vi "VI for temp, humidity, moisture and pH with power supply control final.vi"() -> ()   [LabVIEW 2022 SP3]
uses:
  <vilib>/DAQmx/read.llb/DAQmx Read (Analog 1D DBL NChan 1Samp).vi
  <vilib>/DAQmx/write.llb/DAQmx Write (Digital Bool 1Line 1Point).vi
  <vilib>/DAQmx/create/channels.llb/DAQmx Create Channel (AI-Voltage-Basic).vi
  <vilib>/DAQmx/create/channels.llb/DAQmx Create Channel (DO-Digital Output).vi
  <vilib>/DAQmx/miscellaneous.llb/DAQmx Fill In Error Info.vi
panel:
  out "pH meter":dbl(knob) scale=0.0..14.0
  out "Moisture":dbl(knob) scale=0.0..100.0
  out "Temperature":dbl(knob) scale=0.0..40.0
  out "Humidity":dbl(knob) scale=0.0..100.0
  in  "LED to notify pH level is out of range":tag
  in  "Trigger pump to water the plant":tag
  in  "VISA resource name - for close channel":refnum<visa-resource-name>
  in  "VISA resource name - for open channel":refnum<visa-resource-name>
  in  "Fan to reduce temperature":tag
  in  "Humidifier to increase humidity":tag
  in  "Fan to reduce humidity":tag
  in  "physical channels":tag
  in  "stop":bool
  out "voltage for humidity":dbl
  out "Humidity level":dbl
  out "Temperature level":dbl
  out "voltage for temperature":dbl
  out "voltage for moisture sensor":dbl
  out "voltage for pH level":dbl
  out "Moisture level":dbl
  out "pH level":dbl
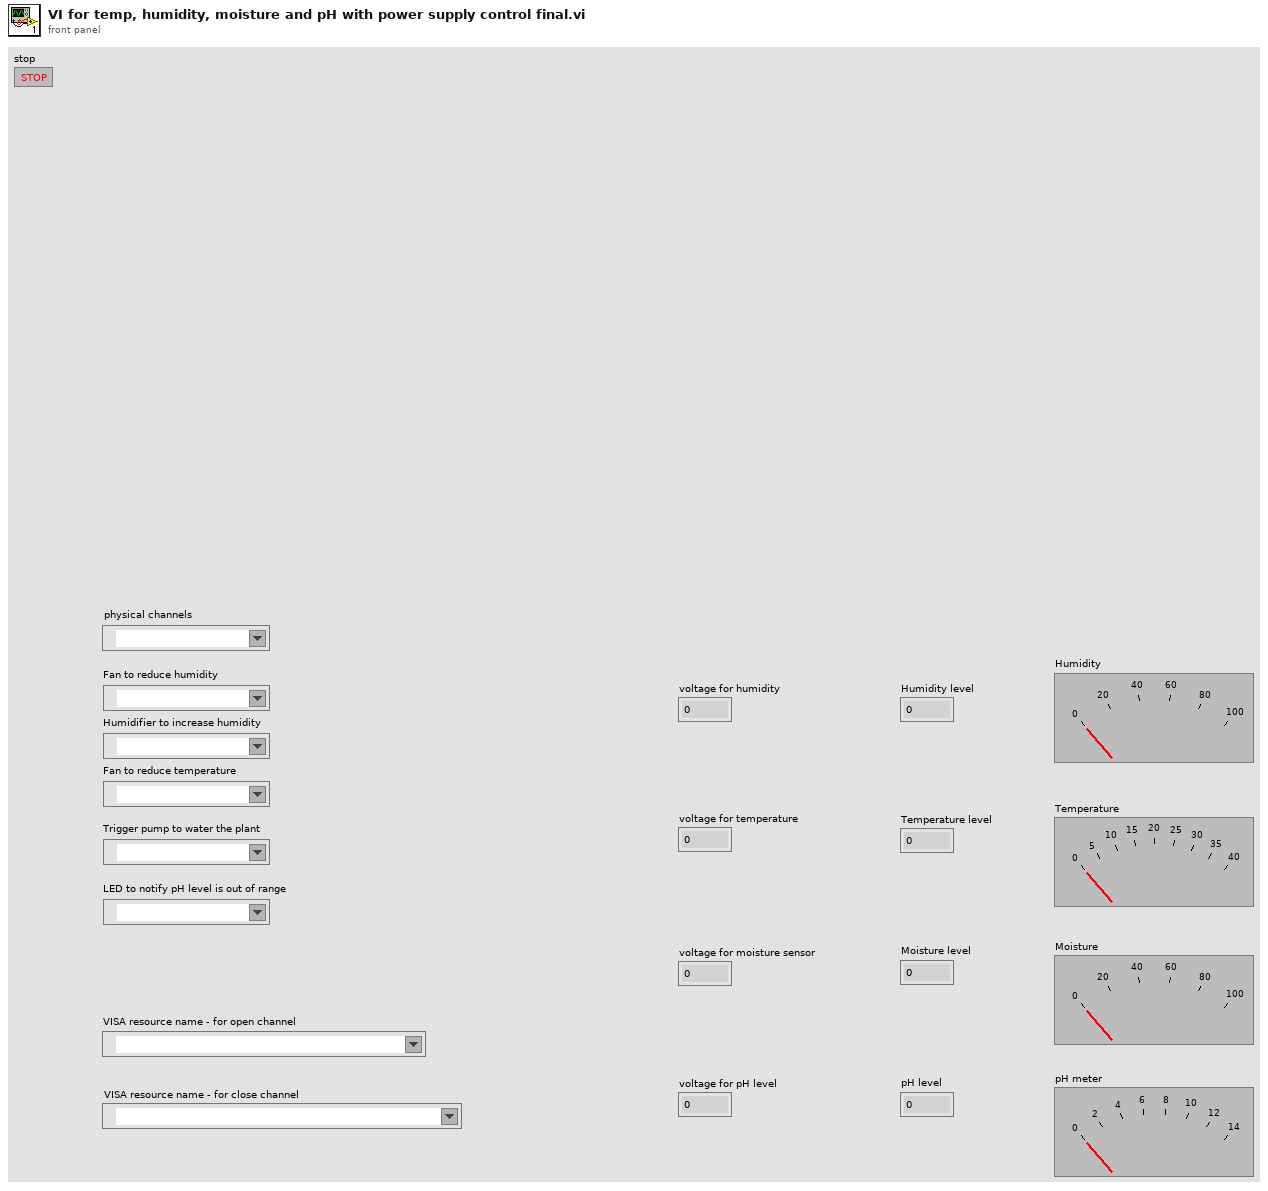
[diagram p1: front panel]
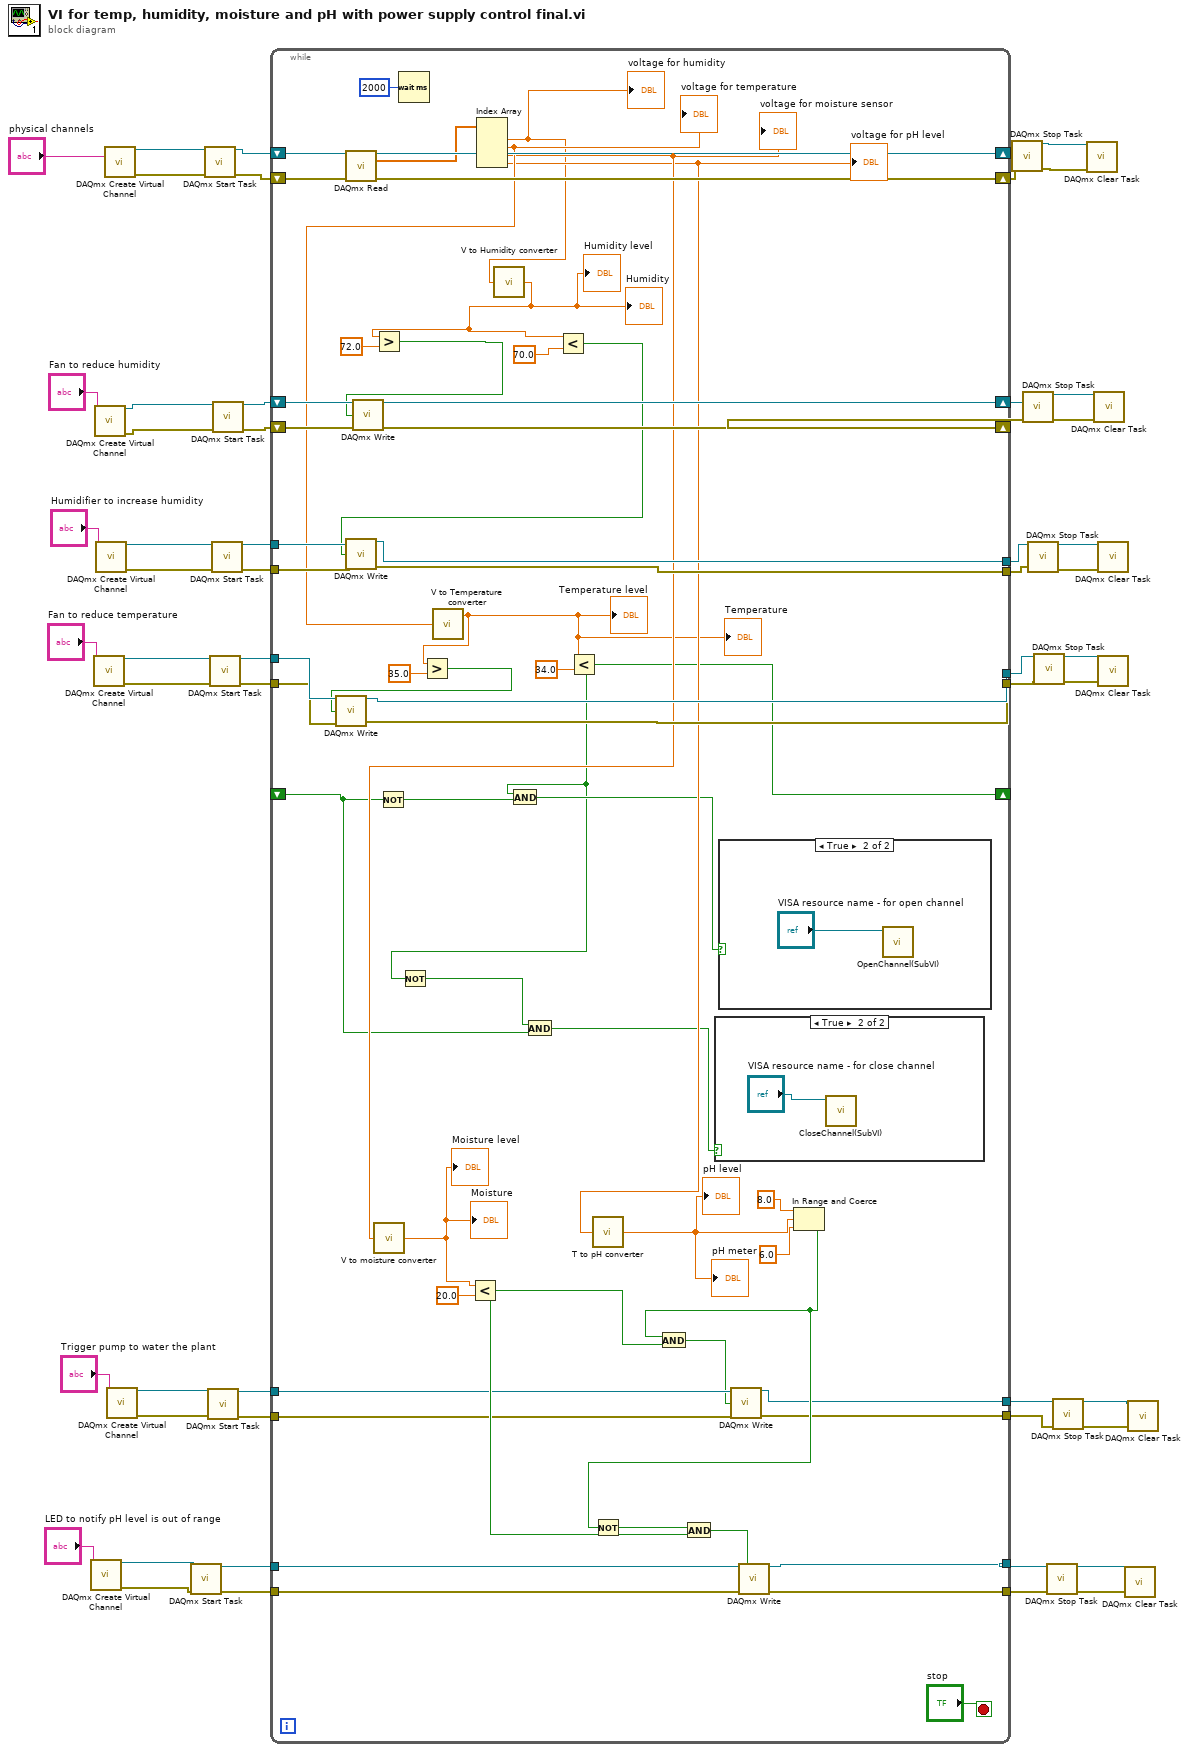
[diagram p0: block diagram]
diagram:
  n1 = call-poly <vilib>:"DAQmx Create Virtual Channel.vi"("lines"="LED to notify pH level is out of range") -> ("task out"=w9:refnum<k21>, "error out"=w5:errorcluster)  [unwired: 13 in]
  n2 = call-poly <vilib>:"DAQmx Create Virtual Channel.vi"("lines"="Fan to reduce temperature") -> ("task out"=w27:refnum<k21>, "error out"=w26:errorcluster)  [unwired: 13 in]
  n3 = call-poly <vilib>:"DAQmx Create Virtual Channel.vi"("lines"="Fan to reduce humidity") -> ("task out"=w46:refnum<k21>, "error out"=w42:errorcluster)  [unwired: 13 in]
  n4 = call-poly <vilib>:"DAQmx Create Virtual Channel.vi"("lines"="Humidifier to increase humidity") -> ("task out"=w36:refnum<k21>, "error out"=w35:errorcluster)  [unwired: 13 in]
  n5 = call-poly <vilib>:"DAQmx Create Virtual Channel.vi"("physical channels"="physical channels") -> ("task out"=w54:refnum<k21>, "error out"=w50:errorcluster)  [unwired: 13 in]
  n6 = call-poly <vilib>:"DAQmx Create Virtual Channel.vi"("lines"="Trigger pump to water the plant") -> ("task out"=w18:refnum<k21>, "error out"=w14:errorcluster)  [unwired: 13 in]
  n7 = call <vilib>:"DAQmx Start Task.vi"("task/channels in"=w9, "error in"=w5) -> ("task out"=w8:refnum<k21>, "error out"=w4:errorcluster)  [unwired: 12 in]
  n8 = call <vilib>:"DAQmx Start Task.vi"("task/channels in"=w54, "error in"=w50) -> ("task out"=w53:refnum<k21>, "error out"=w49:errorcluster)  [unwired: 12 in]
  n9 = call <vilib>:"DAQmx Start Task.vi"("task/channels in"=w18, "error in"=w14) -> ("task out"=w17:refnum<k21>, "error out"=w13:errorcluster)  [unwired: 12 in]
  n10 = call <vilib>:"DAQmx Start Task.vi"("task/channels in"=w27, "error in"=w26) -> ("task out"=w24:refnum<k21>, "error out"=w23:errorcluster)  [unwired: 12 in]
  n11 = call <vilib>:"DAQmx Start Task.vi"("task/channels in"=w36, "error in"=w35) -> ("task out"=w34:refnum<k21>, "error out"=w33:errorcluster)  [unwired: 12 in]
  n12 = call <vilib>:"DAQmx Start Task.vi"("task/channels in"=w46, "error in"=w42) -> ("task out"=w45:refnum<k21>, "error out"=w41:errorcluster)  [unwired: 12 in]
  n13 = while {
    shift-right: [w109] -> w52
    shift-left: w53 -> [w110]
    shift-right: [w107] -> w48
    shift-left: w49 -> [w108]
    shift-right: [w105] -> w44
    shift-left: w45 -> [w106]
    shift-right: [w103] -> w40
    shift-left: w41 -> [w104]
    tunnel: w34 -> [w98]
    tunnel: w33 -> [w97]
    tunnel: [w96] -> w32
    tunnel: [w95] -> w31
    tunnel: w24 -> [w94]
    tunnel: w23 -> [w93]
    tunnel: [w92] -> w22
    tunnel: [w91] -> w21
    shift-right: [w81] -> _
    shift-left: _ -> [w63]
    tunnel: w17 -> [w74]
    tunnel: [w73] -> w16
    tunnel: w13 -> [w72]
    tunnel: [w71] -> w12
    tunnel: w8 -> [w69]
    tunnel: [w68] -> w7
    tunnel: w4 -> [w67]
    tunnel: [w66] -> w3
    stop <- "stop" stop-if-true
    n14 = call-poly <vilib>:"DAQmx Read.vi"("task/channels in"=w110, "error in"=w108) -> ("task out"=w109:refnum<k21>, "data"=w100:dbl[], "error out"=w107:errorcluster)  [unwired: 11 in]
    n15 = Not(x=w63) -> (.not. x?=w64:bool)
    n16 = Wait (ms)(milliseconds to wait=u32 2000) -> ()  [unwired: 1 out]
    n17 = Index Array(array=w100) -> (element #1=w78:dbl, element #2=w90:dbl, element #3=w86:dbl, element #4=w83:dbl)  [unwired: 4 in]
    "voltage for humidity" <- w78
    "voltage for temperature" <- w90
    "voltage for moisture sensor" <- w86
    "voltage for pH level" <- w83
    n18 = call "V to moisture converter.vi"("Waveform"=w86) -> ("Numeric"=w56:dbl)
    "Moisture level" <- w56
    "Moisture" <- w56
    n19 = call "V to Temperature converter.vi"("Waveform"=w90) -> ("Numeric"=w57:dbl)
    "Temperature level" <- w57
    "Temperature" <- w57
    n20 = Greater?(x=w57, y=35.0) -> (0:w59:bool)
    n21 = call-poly <vilib>:"DAQmx Write.vi"("task/channels in"=w94, "data"=w59, "error in"=w93) -> ("task out"=w92:refnum<k21>, "error out"=w91:errorcluster)  [unwired: 10 in, 1 out]
    n22 = Less?(x=w56, y=20.0) -> (x < y?=w75:bool)
    n23 = call "V to Humidity converter.vi"("Waveform"=w78) -> ("Numeric"=w58:dbl)
    "Humidity level" <- w58
    "Humidity" <- w58
    n24 = Greater?(x=w58, y=72.0) -> (0:w60:bool)
    n25 = call-poly <vilib>:"DAQmx Write.vi"("task/channels in"=w106, "data"=w60, "error in"=w104) -> ("task out"=w105:refnum<k21>, "error out"=w103:errorcluster)  [unwired: 10 in, 1 out]
    n26 = Less?(x=w58, y=70.0) -> (x < y?=w61:bool)
    n27 = call-poly <vilib>:"DAQmx Write.vi"("task/channels in"=w98, "data"=w61, "error in"=w97) -> ("task out"=w96:refnum<k21>, "error out"=w95:errorcluster)  [unwired: 10 in, 1 out]
    n28 = Less?(x=w57, y=34.0) -> (x < y?=w81:bool)
    n29 = Not(x=w81) -> (.not. x?=w80:bool)
    n30 = And(x=w81, y=w64) -> (x .and. y?=w82:bool)
    n31 = And(x=w80, y=w63) -> (x .and. y?=w79:bool)
    n32 = call "T to pH converter.vi"("Waveform"=w83) -> ("Numeric"=w55:dbl)
    "pH level" <- w55
    "pH meter" <- w55
    n33 = case shown="True" w79 {
      frame False {
      }
      frame True {
        n34 = call "CloseChannel(SubVI).vi"("VISA Refnum in"="VISA resource name - for close channel") -> ()  [unwired: 11 in]
      }
    }
    n35 = case shown="True" w82 {
      frame False {
      }
      frame True {
        n36 = call "OpenChannel(SubVI).vi"("VISA Refnum in"="VISA resource name - for open channel") -> ()  [unwired: 11 in]
      }
    }
    n37 = In Range and Coerce(upper limit=8.0, x=w55, lower limit=6.0) -> (In Range?=w77:bool)  [unwired: 1 out]
    n38 = Not(x=w77) -> (.not. x?=w76:bool)
    n39 = And(x=w77, y=w75) -> (x .and. y?=w70:bool)
    n40 = And(x=w76, y=w75) -> (x .and. y?=w65:bool)
    n41 = call-poly <vilib>:"DAQmx Write.vi"("task/channels in"=w74, "data"=w70, "error in"=w72) -> ("task out"=w73:refnum<k21>, "error out"=w71:errorcluster)  [unwired: 10 in, 1 out]
    n42 = call-poly <vilib>:"DAQmx Write.vi"("task/channels in"=w69, "data"=w65, "error in"=w67) -> ("task out"=w68:refnum<k21>, "error out"=w66:errorcluster)  [unwired: 10 in, 1 out]
  }
  n43 = call <vilib>:"DAQmx Stop Task.vi"("task/channels in"=w52, "error in"=w48) -> ("task out"=w51:refnum<k21>, "error out"=w47:errorcluster)  [unwired: 12 in]
  n44 = call <vilib>:"DAQmx Stop Task.vi"("task/channels in"=w44, "error in"=w40) -> ("task out"=w43:refnum<k21>, "error out"=w39:errorcluster)  [unwired: 12 in]
  n45 = call <vilib>:"DAQmx Stop Task.vi"("task/channels in"=w32, "error in"=w31) -> ("task out"=w30:refnum<k21>, "error out"=w29:errorcluster)  [unwired: 12 in]
  n46 = call <vilib>:"DAQmx Stop Task.vi"("task/channels in"=w22, "error in"=w21) -> ("task out"=w20:refnum<k21>, "error out"=w19:errorcluster)  [unwired: 12 in]
  n47 = call <vilib>:"DAQmx Stop Task.vi"("task/channels in"=w7, "error in"=w3) -> ("task out"=w6:refnum<k21>, "error out"=w2:errorcluster)  [unwired: 12 in]
  n48 = call <vilib>:"DAQmx Stop Task.vi"("task/channels in"=w16, "error in"=w12) -> ("task out"=w15:refnum<k21>, "error out"=w11:errorcluster)  [unwired: 12 in]
  n49 = call <vilib>:"DAQmx Clear Task.vi"("task in"=w51, "error in"=w47) -> ()  [unwired: 13 in, 1 out]
  n50 = call <vilib>:"DAQmx Clear Task.vi"("task in"=w43, "error in"=w39) -> ()  [unwired: 13 in, 1 out]
  n51 = call <vilib>:"DAQmx Clear Task.vi"("task in"=w30, "error in"=w29) -> ()  [unwired: 13 in, 1 out]
  n52 = call <vilib>:"DAQmx Clear Task.vi"("task in"=w20, "error in"=w19) -> ()  [unwired: 13 in, 1 out]
  n53 = call <vilib>:"DAQmx Clear Task.vi"("task in"=w6, "error in"=w2) -> ()  [unwired: 13 in, 1 out]
  n54 = call <vilib>:"DAQmx Clear Task.vi"("task in"=w15, "error in"=w11) -> ()  [unwired: 13 in, 1 out]
